vi "Calculate Makespan.vi"() -> ()   [LabVIEW 2013]
uses:
  Classes/GanntChart.lvclass
panel:
  out "Machine Completion Times":u16[](array[numeric])
  out "Job Completion Times":u16[](array[numeric])
  out "max value":u16
  in  "Number of  Jobs":i32=4
  in  "Number of Machines":i32=4
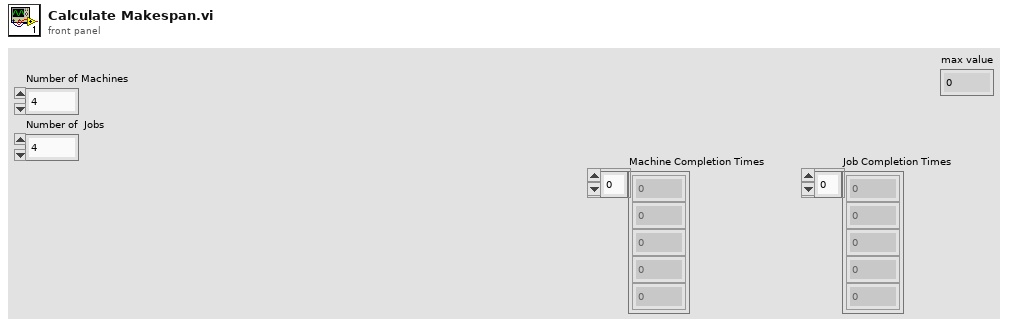
[diagram p1: front panel]
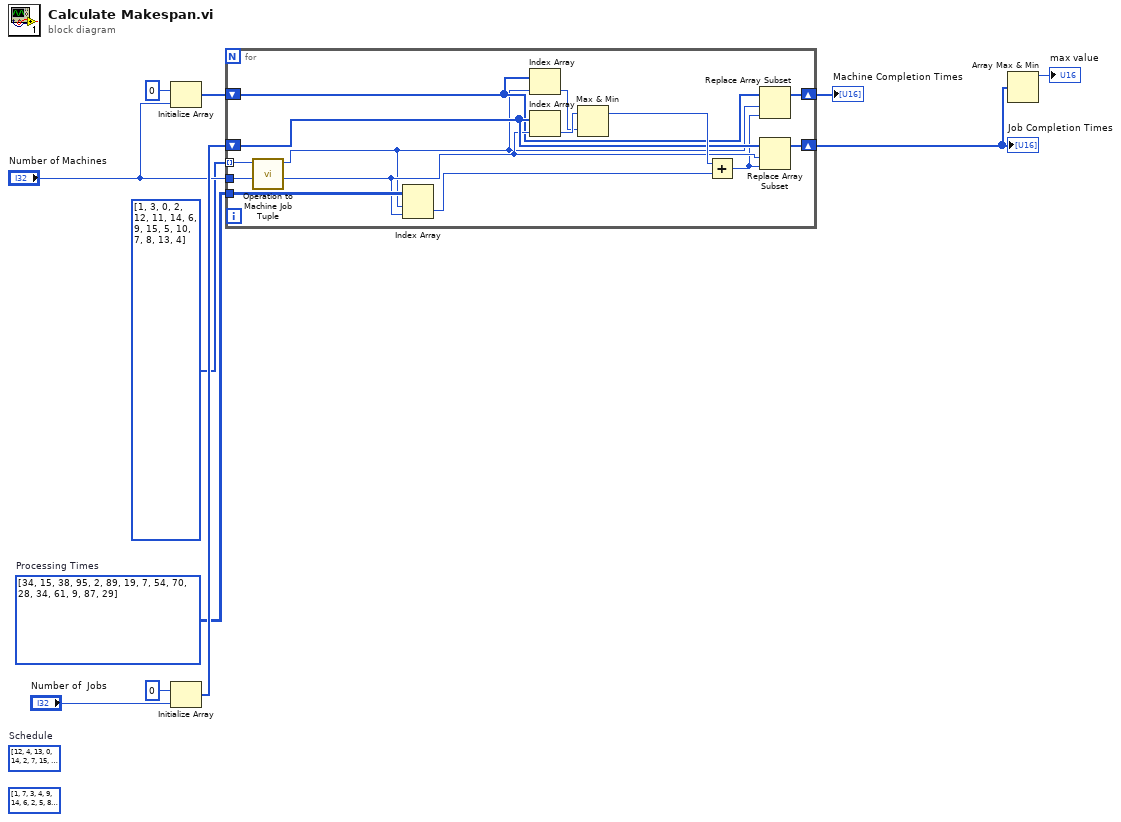
[diagram p0: block diagram]
diagram:
  (unwired) u16[] [1, 7, 3, 4, 9, 14, 6, 2, 5, 8, 13, 11, 0, 12, 10, 15] ("Schedule")
  w7 = u16[][] [[34, 15, 38, 95], [2, 89, 19, 7], [54, 70, 28, 34], [61, 9, 87, 29]]  # Processing Times
  (unwired) u16[] [12, 4, 13, 0, 14, 2, 7, 15, 9, 1, 6, 3, 11, 10, 5, 8]  # Schedule
  n1 = Initialize Array(u16 0 ("element"), "Number of Machines") -> (w8:u16[])
  n2 = Initialize Array(u16 0 ("element"), "Number of  Jobs") -> (w9:u16[])
  n3 = for {
    tunnel: "Number of Machines" -> [w24]
    shift-right: [w12] -> w4
    shift-left: w9 -> [w18]
    shift-right: [w13] -> w2
    shift-left: w8 -> [w16]
    tunnel: w7 -> [w21]
    tunnel: u16[] [1, 3, 0, 2, 12, 11, 14, 6, 9, 15, 5, 10, 7, 8, 13, 4] -> [w25] mode=indexing
    n4 = call "Operation to Machine Job Tuple.vi"("Number of Machines"=w24, "Operation Number"=w25) -> ("Job No"=w17:i32, "Machine No"=w15:i32)  [unwired: 8 in]
    n5 = Index Array(array=w21, index (row)=w15, index (col)=w17) -> (element=w19:u16)
    n6 = Index Array(array=w16, index=w15) -> (element=w22:u16)
    n7 = Index Array(array=w18, index=w17) -> (element=w23:u16)
    n8 = Max & Min(x=w23, y=w22) -> (max(x,y)=w20:u16)  [unwired: 1 out]
    n9 = Add(x=w20, y=w19) -> (x+y=w14:u16)
    n10 = Replace Array Subset(array=w16, new element=w14, index=w15) -> (w13:u16[])
    n11 = Replace Array Subset(array=w18, new element=w14, index=w17) -> (w12:u16[])
  }
  "Job Completion Times" <- w4
  "Machine Completion Times" <- w2
  n12 = Array Max & Min(array=w4) -> (max value=→"max value":u16)  [unwired: 3 out]
